vi "Transmit Scheduled and Dynamic Messages.vi"() -> ()   [LabVIEW 2019]
doc: "This example program opens the specified card and core, configures a transmit \nchannel with one scheduled message, and creates an asynchronous transmit list\n buffer. The program transmits one label synchronously in a schedule, and \ntransmits another label each time the Async button is pressed."
uses:
  <instrlib>/BTICardLib/Private/Initialize By Card Number and Core Number.vi
  <instrlib>/BTICardLib/Private/Configure Core From XML.vi
  <instrlib>/BTI429Lib/Private/Tx/Configure/Configure Tx Channel From XML.vi
  <instrlib>/BTI429Lib/Private/Core/Action-Status/Start All Channels.vi
  <instrlib>/BTI429Lib/Private/Tx/Data/Transmit Message Dynamic.vi
  <instrlib>/BTI429Lib/Private/Core/Action-Status/Stop All Channels.vi
  <instrlib>/BTI429Lib/BTI429LV.lvlib
  <instrlib>/BTICardLib/BTICardLV.lvlib
panel:
  out "core number":i32
  out "channel number":i32
  out "Async Message Count":u32
  in  "Send Asynchronous Message":bool
  out "error out":errorcluster
  in  "stop":bool
  in  "Channel XML Configuration":string="Channel Config.xml"
  in  "Core XML Configuration":string="Core Config.xml"
  in  "Card Number":i32
  # "ARINC 429: Transmit Scheduled and Dynamic Messages"
  # "©2016 Astronics Ballard Technology"
  # "This example program opens the specified card and core, configures a transmit \nchannel with one scheduled message, and creates an asynchronous transmit list\n buffer. The program transmits one label synchronously in a schedule, and \ntransmits another label each time the Async button is pressed."
  # "Always Stop the card\nand Close the card when\ndone. Otherwise, the hardware\ncontinues to operate."
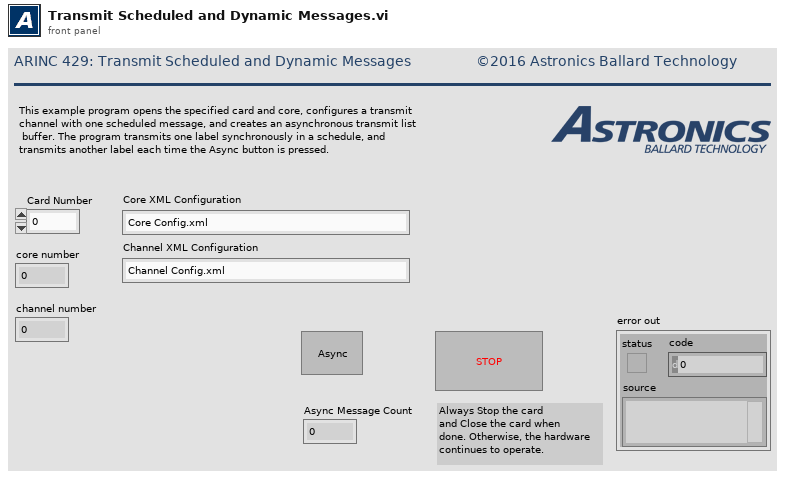
[diagram p1: front panel]
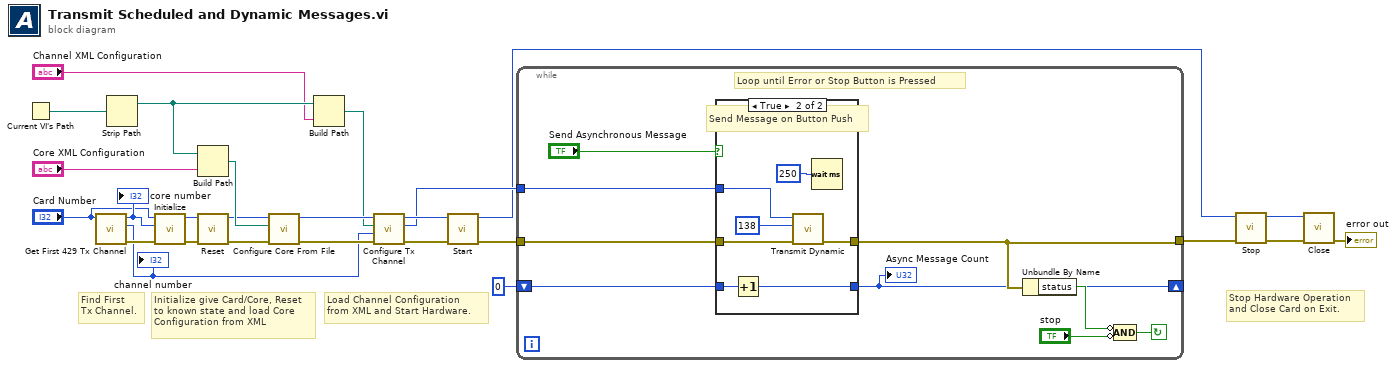
[diagram p0: block diagram]
diagram:
  # "Find First\nTx Channel."
  # "Load Channel Configuration\nfrom XML and Start Hardware."
  # "Initialize give Card/Core, Reset\nto known state and load Core\nConfiguration from XML"
  # "Stop Hardware Operation\nand Close Card on Exit."
  n1 = Current VI's Path() -> (path=w20:path)
  n2 = call "Get First 429 Tx Channel.vi"("Card Number"="Card Number") -> ("error out"=w2:errorcluster, "Channel Number"=w1:i32, "Core Number"=w4:i32)  [unwired: 8 in]
  "channel number" <- w1
  "core number" <- w4
  n3 = Strip Path(path=w20) -> (stripped path=w19:path)  [unwired: 1 out]
  n4 = call-poly <instrlib>:"Initialize.vi"("error in (no error)"=w2, "core number"=w4, "card number"="Card Number") -> ("error out"=w7:errorcluster, "core handle out"=w8:u64)  [unwired: 7 in]
  n5 = Build Path(base path=w19, name or relative path="Core XML Configuration") -> (appended path=w17:path)
  n6 = call <instrlib>:"Reset.vi"("error in (no error)"=w7, "core handle in"=w8) -> ("error out"=w6:errorcluster, "core handle out"=w9:u64)  [unwired: 8 in]
  n7 = call-poly <instrlib>:"Configure Core From File.vi"("error in (no error)"=w6, "configuration file path"=w17, "core handle in"=w9) -> ("error out"=w25:errorcluster, "core handle out"=w26:u64)  [unwired: 7 in]
  n8 = Build Path(base path=w19, name or relative path="Channel XML Configuration") -> (appended path=w15:path)
  n9 = call-poly <instrlib>:"Configure Tx Channel.vi"("error in (no error)"=w25, "channel number in"=w1, "configuration file path"=w15, "core handle in"=w26) -> ("error out"=w23:errorcluster, "channel handle out"=w14:u64, "core handle out"=w22:u64)  [unwired: 5 in]
  n10 = call-poly <instrlib>:"Start.vi"("error in (no error)"=w23, "core handle in"=w22) -> ("error out"=w24:errorcluster, "core handle out"=w10:u64)  [unwired: 8 in]
  n11 = while {
    tunnel: w14 -> [w32]
    tunnel: w24 -> [w31]
    tunnel: [w30] -> w12
    shift-right: [w27] -> _
    shift-left: u32 0 -> [w28]
    stop <- w34 continue-if-true
    # "Loop until Error or Stop Button is Pressed"
    n12 = case shown="True" "Send Asynchronous Message" {
      tunnel: w32 -> [_ w44]
      tunnel: [w36 w43] -> w27
      tunnel: w28 -> [w36 w42]
      tunnel: w31 -> [w37 w40]
      tunnel: [w37 w39] -> w30
      frame False {
      }
      frame True {
        # "Send Message on Button Push"
        n13 = Increment(x=w42) -> (x+1=w43:u32)
        n14 = call-poly <instrlib>:"Transmit Dynamic.vi"("error in (no error)"=w40, "message data"=u32 138 ("y"), "channel handle in"=w44) -> ("error out"=w39:errorcluster)  [unwired: 7 in, 1 out]
        n15 = Wait (ms)(milliseconds to wait=u32 250) -> ()  [unwired: 1 out]
      }
    }
    "Async Message Count" <- w27
    n16 = Unbundle By Name(w30) -> ("status"=w29:bool)
    n17 = Compound Arithmetic op=AND(invert w29, invert "stop") -> (w34:bool)
  }
  n18 = call-poly <instrlib>:"Stop.vi"("error in (no error)"=w12, "core handle in"=w10) -> ("error out"=w13:errorcluster, "core handle out"=w11:u64)  [unwired: 8 in]
  n19 = call <instrlib>:"Close.vi"("error in (no error)"=w13, "core handle in"=w11) -> ("error out"=→"error out":errorcluster)  [unwired: 8 in, 1 out]
